vi "lines_number.vi"(1 "file path":path) -> (0 "No. lines":i32)   [LabVIEW 2018]
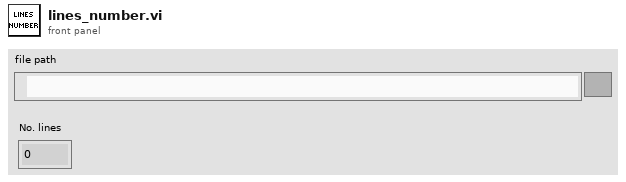
[diagram p1: front panel]
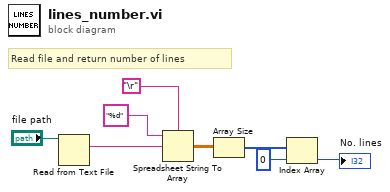
[diagram p0: block diagram]
diagram:
  # "Read file and return number of lines"
  n1 = Read from Text File(file (use dialog)="file path") -> (text=w5:string)  [unwired: 3 in, 3 out]
  n2 = Spreadsheet String To Array(delimiter (Tab)="\r", format string="%d", spreadsheet string=w5) -> (array=w6:dbl[][])  [unwired: 1 in]
  n3 = Array Size(array=w6) -> (size(s)=w2:i32[])
  n4 = Index Array(array=w2, index=0) -> (element=→"No. lines":i32)
